vi "filter_logic_chargeupdate.vi"(9 "Filter Specific Constants":T2, 10 "Variables Cluster":T4, 11 "constants cluster":T1={"High Charge Limit"=0, "Low Charge Limit"=0, "Low Velocity Count"=0, "High Velocity Count"=0, "Low Velocity Count"=0, 26666666.59375, "High Mass Limit"=0, "Low Mass Limit"=0}) -> (3 "Output Cluster":T3)   [LabVIEW 2012]
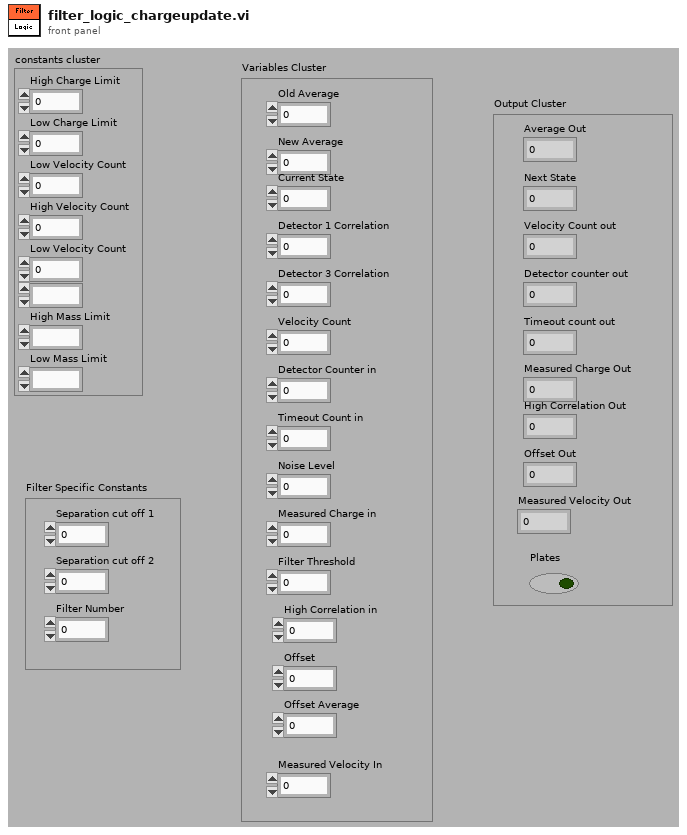
[diagram p1: front panel]
types:
  T1 = cluster{"High Charge Limit":i16, "Low Charge Limit":i16, "Low Velocity Count":i32, "High Velocity Count":i32, "Low Velocity Count":i32, fxp<+,30,25>, "High Mass Limit":i64, "Low Mass Limit":i64}
  T2 = cluster{"Separation cut off 1":i32, "Filter Number":i32, "Separation cut off 2":i32}
  T3 = cluster{"Average Out":i32, "Next State":u8, "Velocity Count out":i32, "Detector counter out":i32, "Timeout count out":u32, "Measured Charge Out":i32, "High Correlation Out":i32, "Plates":bool, "Offset Out":i32, "Measured Velocity Out":i32}
  T4 = cluster{"Old Average":i32, "New Average":i32, "Current State":u8, "Detector 1 Correlation":i32, "Detector 3 Correlation":i32, "Velocity Count":i32, "Detector Counter in":i32, "Timeout Count in":i32, "Noise Level":i32, "Measured Charge in":i32, "Filter Threshold":i32, "High Correlation in":i32, "Offset":i32, "Offset Average":i32, "Measured Velocity In":i32}
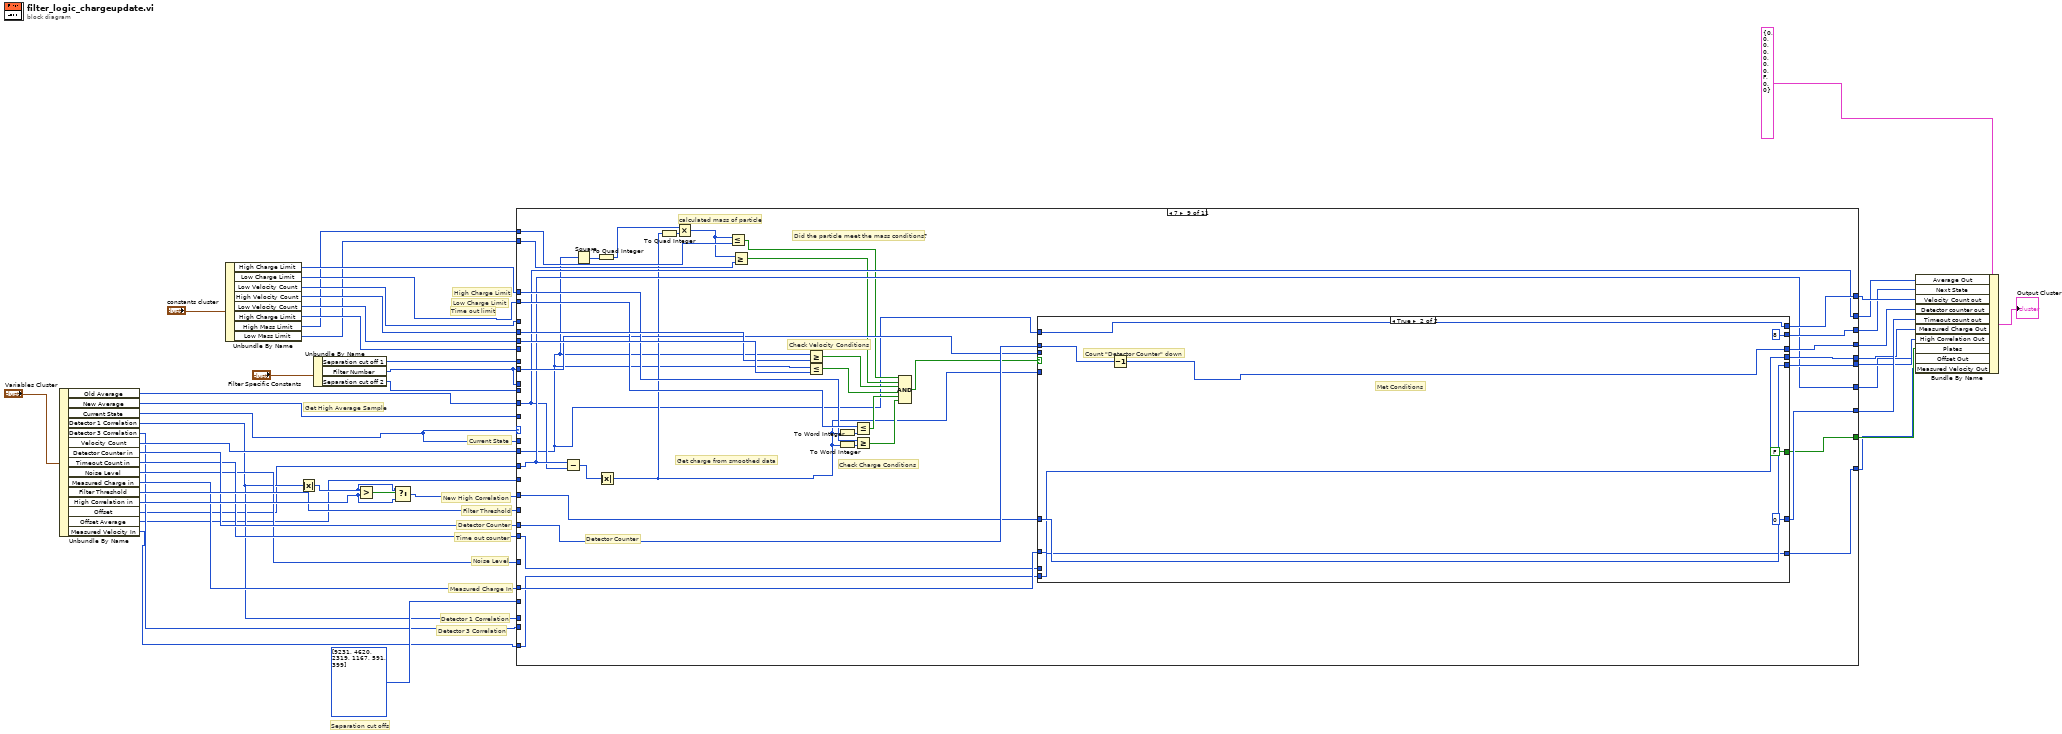
[diagram p0: block diagram]
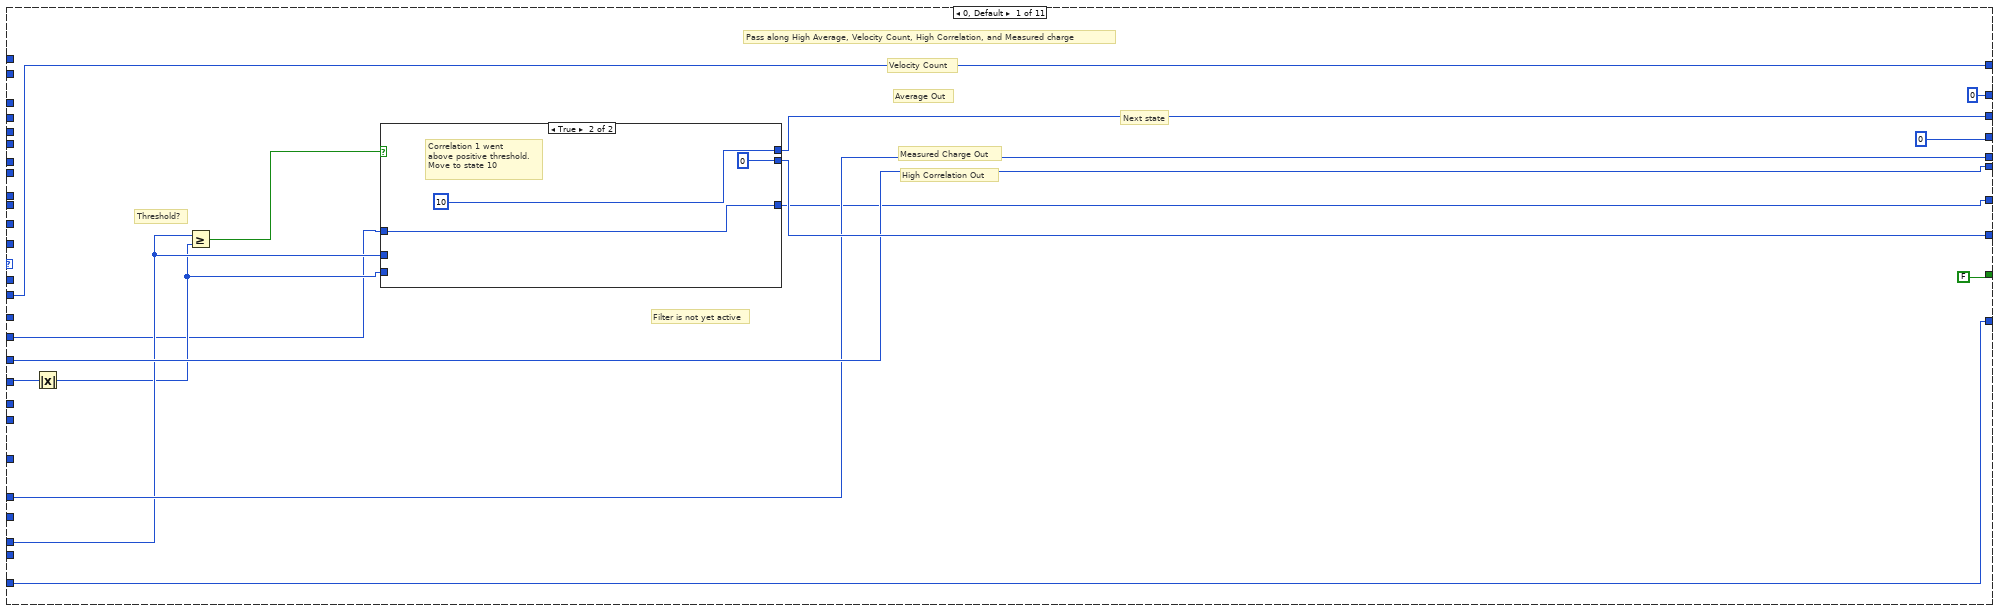
[diagram p2: hidden frame]
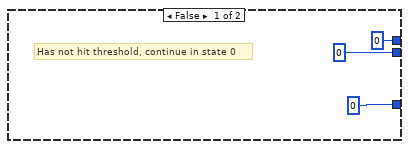
[diagram p3: hidden frame]
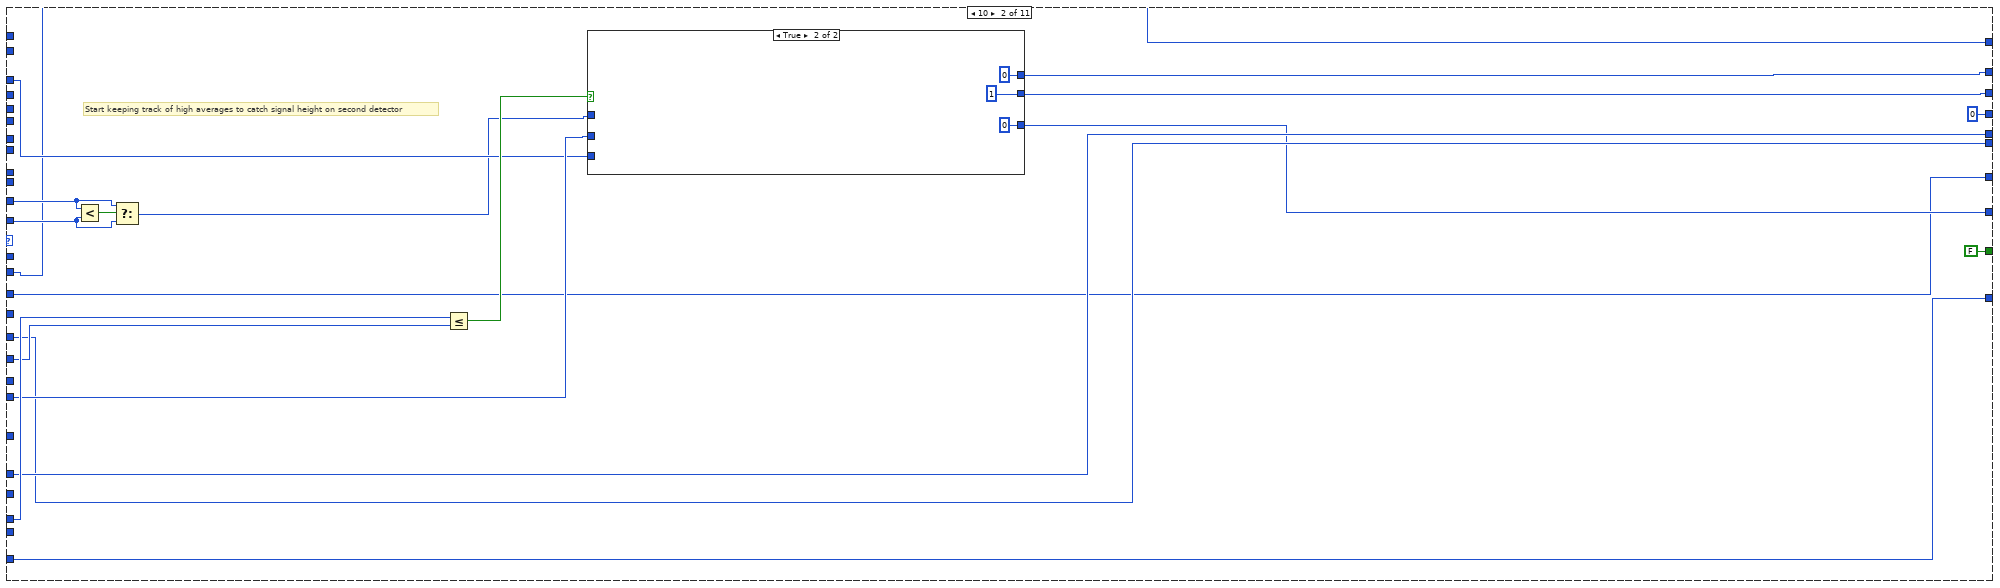
[diagram p4: hidden frame]
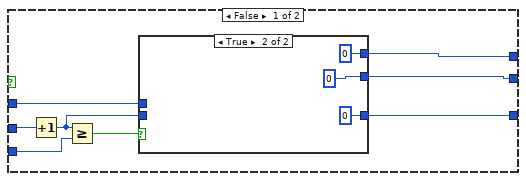
[diagram p5: hidden frame]
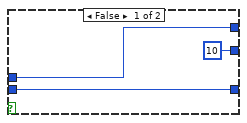
[diagram p6: hidden frame]
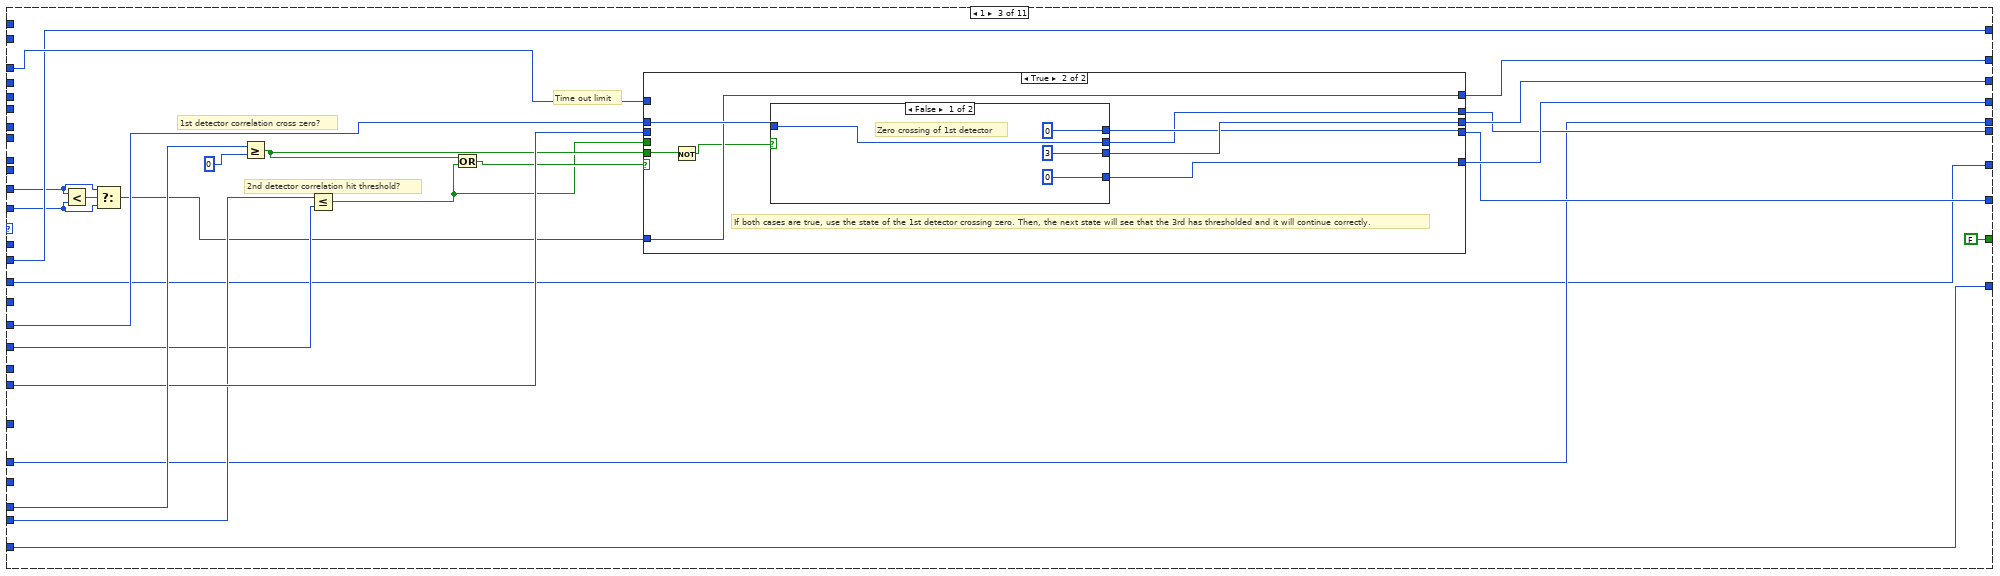
[diagram p7: hidden frame]
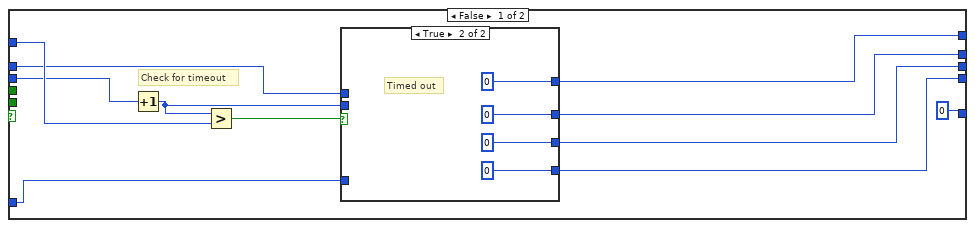
[diagram p8: hidden frame]
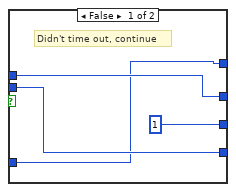
[diagram p9: hidden frame]
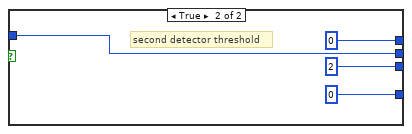
[diagram p10: hidden frame]
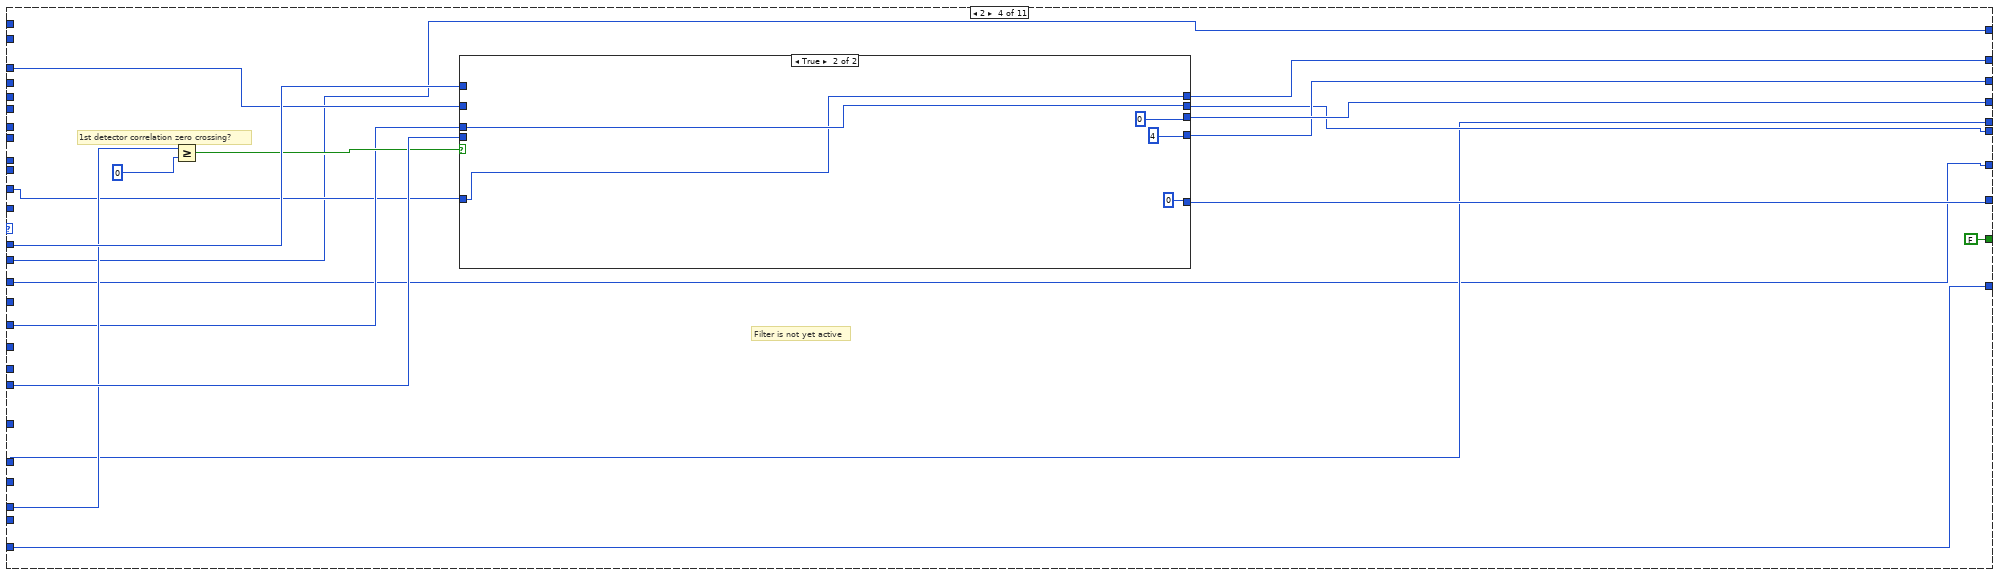
[diagram p11: hidden frame]
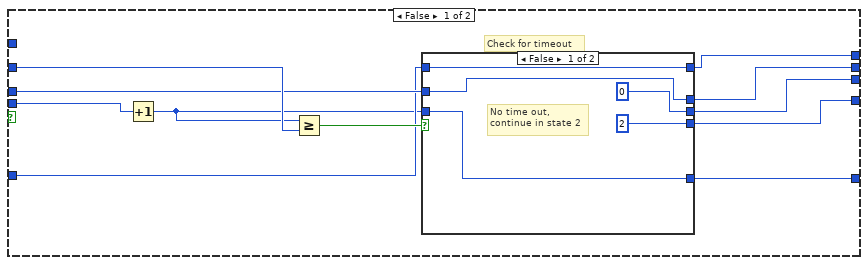
[diagram p12: hidden frame]
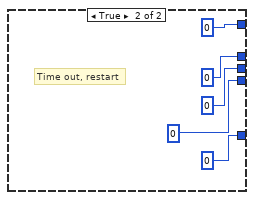
[diagram p13: hidden frame]
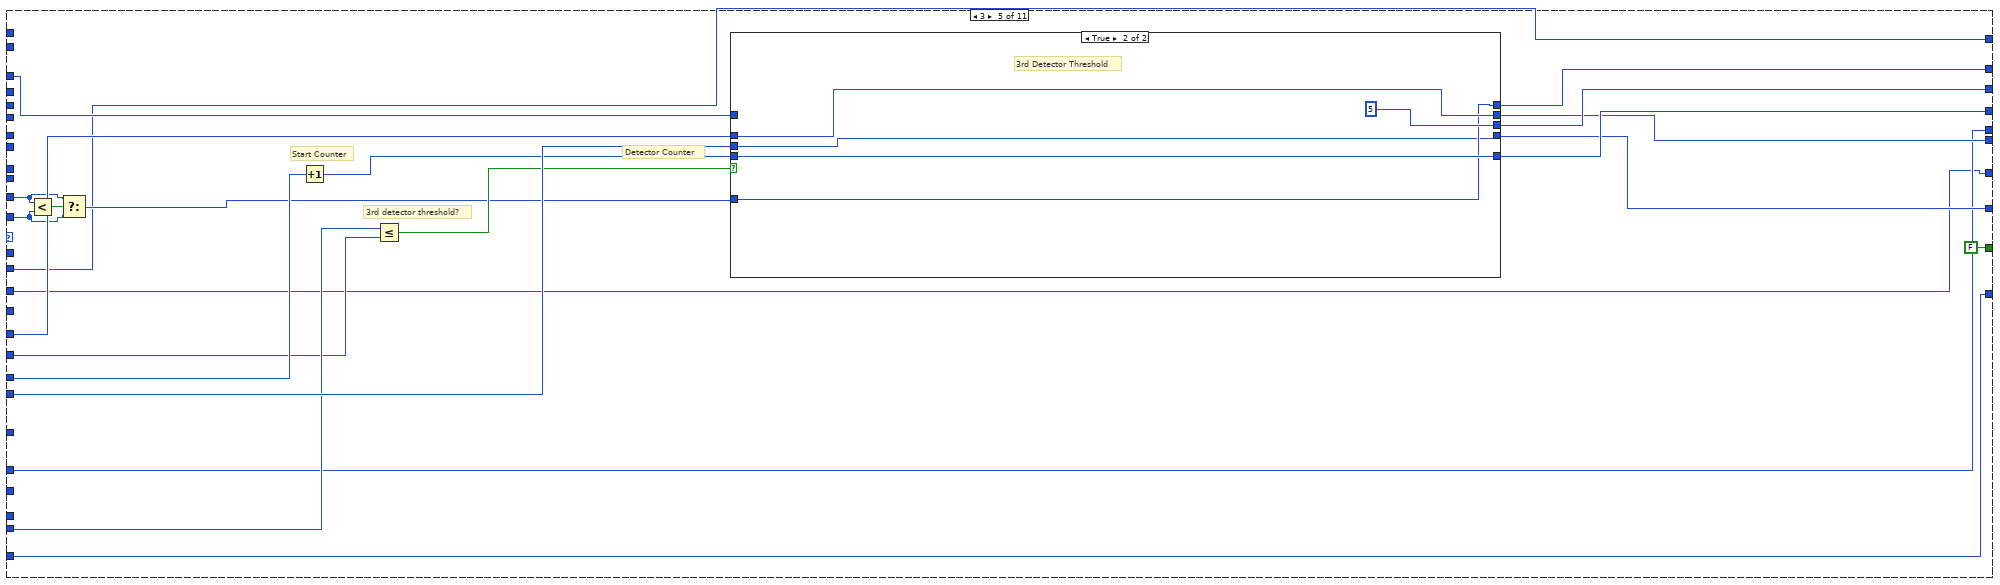
[diagram p14: hidden frame]
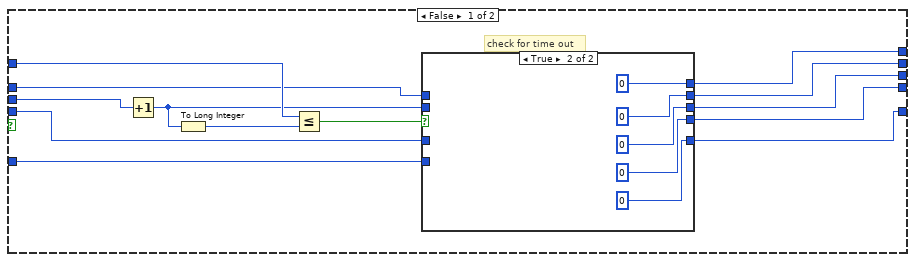
[diagram p15: hidden frame]
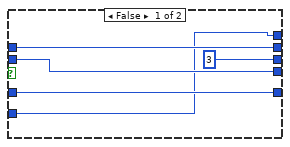
[diagram p16: hidden frame]
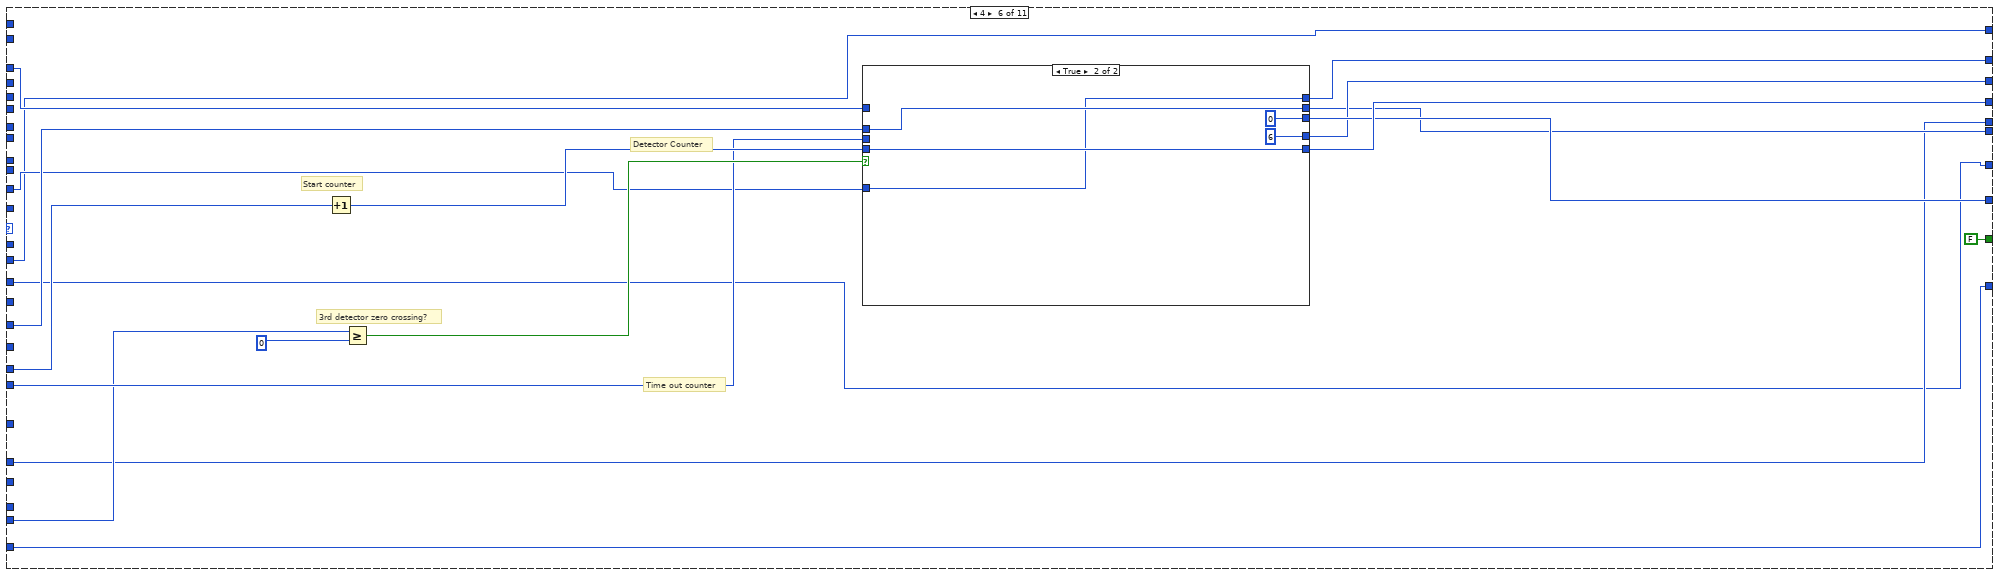
[diagram p17: hidden frame]
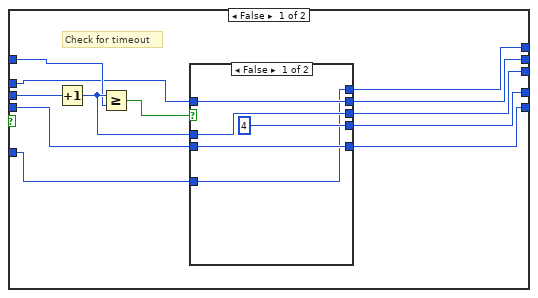
[diagram p18: hidden frame]
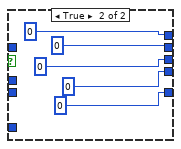
[diagram p19: hidden frame]
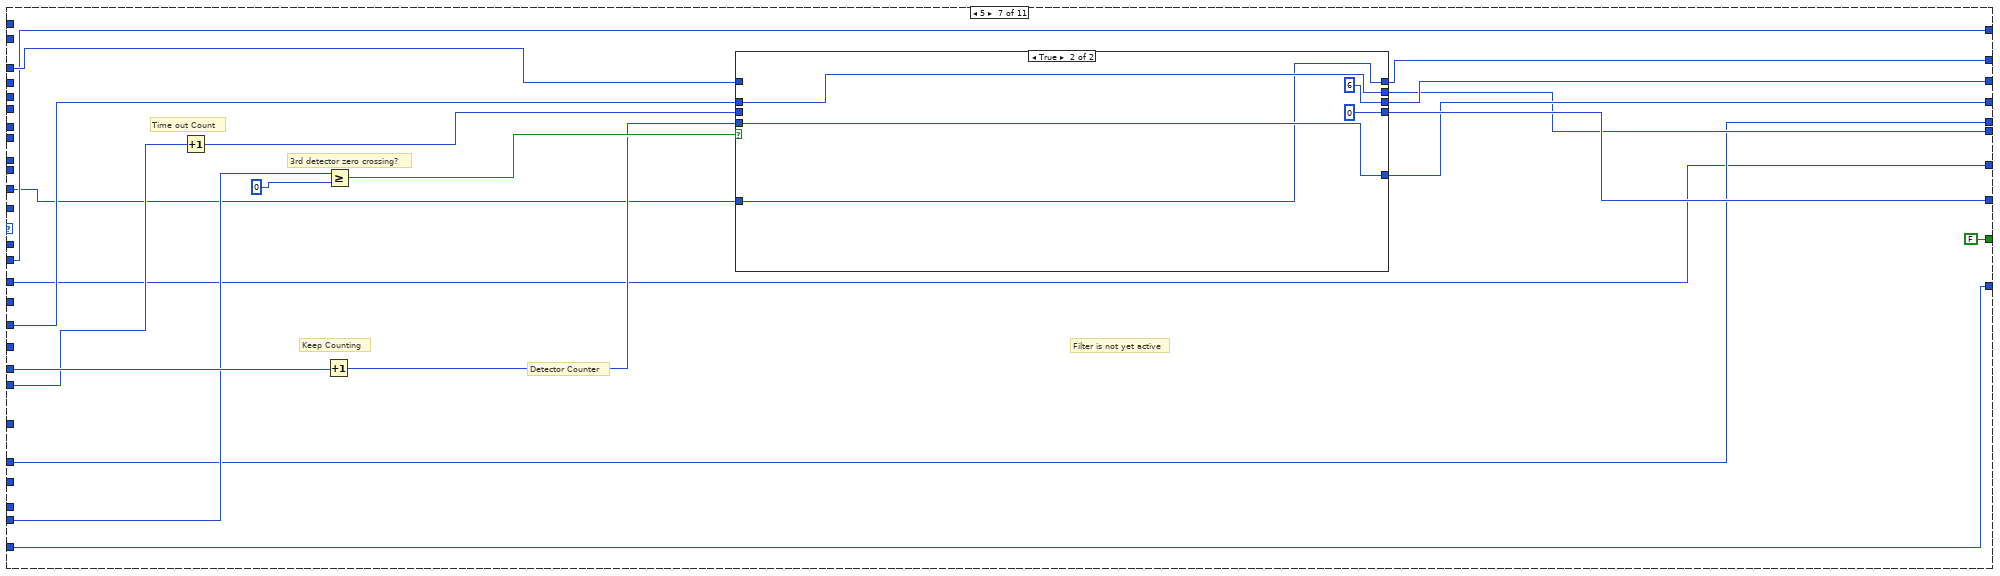
[diagram p20: hidden frame]
diagram:
  # "Detector 3 Correlation"
  # "Detector 1 Correlation"
  # "Separation cut offs"
  # "Measured Charge In"
  # "Noise Level"
  # "Time out counter"
  # "Detector Counter"
  # "Filter Threshold"
  # "New High Correlation"
  # "Current State"
  # "Get High Average Sample"
  # "Time out limit"
  # "Low Charge Limit"
  # "High Charge Limit"
  n1 = Unbundle By Name("Variables Cluster") -> ("Old Average"=w17:i32, "New Average"=w16:i32, "Current State"=w39:u8, "Detector 1 Correlation"=w27:i32, "Detector 3 Correlation"=w26:i32, "Velocity Count"=w38:i32, "Detector Counter in"=w32:i32, "Timeout Count in"=w31:i32, "Noise Level"=w30:i32, "Measured Charge in"=w29:i32, "Filter Threshold"=w33:i32, "High Correlation in"=w34:i32, "Offset"=w15:i32, "Offset Average"=w14:i32, "Measured Velocity In"=w10:i32)
  n2 = Unbundle By Name("constants cluster") -> ("High Charge Limit"=w9:i16, "Low Charge Limit"=w8:i16, "Low Velocity Count"=w7:i32, "High Velocity Count"=w6:i32, "Low Velocity Count"=w5:i32, "High Charge Limit"=w4:i16, "High Mass Limit"=w3:i64, "Low Mass Limit"=w2:i64)
  n3 = Absolute Value(x=w27) -> (abs(x)=w35:i32)
  n4 = Unbundle By Name("Filter Specific Constants") -> ("Separation cut off 1"=w43:i32, "Filter Number"=w42:i32, "Separation cut off 2"=w41:i32)
  n5 = Greater?(x=w35, y=w34) -> (0:w36:bool)
  n6 = Select(t=w35, s=w36, f=w34) -> (s? t:f=w37:i32)
  n7 = case shown="7" w39 {
    tunnel: w27 -> [w52 w82 w126 w173 _ _ _ _ _ _ _]
    tunnel: w26 -> [_ _ w115 _ w219 w266 w311 _ _ _ _]
    tunnel: w33 -> [w50 w81 w114 _ w218 _ _ _ _ _ _]
    tunnel: w32 -> [_ _ _ _ w221 w274 w320 w354 w482 w515 w549]
    tunnel: [0 0 w124 w179 w227 w272 w313 w366 w481 w511 w545] -> w23
    tunnel: [w60 w79 w123 w178 w226 w269 w316 w363 w480 w513 w546] -> w19
    tunnel: w39 -> [_ _ _ w177 _ _ _ _ _ _ _]
    tunnel: w38 -> [w56 w74 w116 w163 w207 w257 w312 w364 w445 w516 w543]
    tunnel: w7 -> [_ w77 w122 w176 w224 w267 w317 _ _ _ _]
    tunnel: w31 -> [_ w78 w121 w175 w225 w268 w319 _ w469 _ _]
    tunnel: [w59 w69 w120 w174 w223 w270 w315 u32 0 w468 u32 0 ("Timeout Count in") u32 0] -> w22
    tunnel: w5 -> [_ _ _ _ _ _ _ _ w479 _ _]
    tunnel: w6 -> [_ _ _ _ _ _ _ _ w478 _ _]
    tunnel: [w56 w74 w116 w163 w207 w257 w312 w365 w477 w512 w543] -> w25
    tunnel: i32[] [9231, 4620, 2319, 1167, 591, 399] -> [_ _ _ _ _ _ _ w357 _ _ _]
    tunnel: w8 -> [_ _ _ _ _ _ _ _ w476 _ _]
    tunnel: w9 -> [_ _ _ _ _ _ _ _ w475 _ _]
    tunnel: w37 -> [w55 w71 w113 w170 w217 w260 w309 w361 w474 w509 w541]
    tunnel: w30 -> [_ _ _ _ _ _ _ _ _ _ _]
    tunnel: [w55 w71 w112 w169 w216 w264 w308 w362 w473 w509 w542] -> w20
    tunnel: w29 -> [w54 w72 w111 w168 w215 w263 w307 w360 w472 w504 w537]
    tunnel: [w54 w72 w111 w168 w215 w263 w307 w360 w471 w505 w537] -> w21
    tunnel: [0 ("Old Average In") w75 w110 w167 w214 w262 w306 w359 w459 w501 0 ("Old Average In")] -> w24
    tunnel: w43 -> [_ _ _ _ _ _ _ w356 _ _ _]
    tunnel: w42 -> [_ _ _ _ _ _ _ w358 _ _ _]
    tunnel: w42 -> [_ _ _ _ _ _ _ w352 w470 w514 w540]
    tunnel: w41 -> [_ _ _ _ _ _ _ w355 _ _ _]
    tunnel: [FALSE FALSE ("Data") FALSE FALSE FALSE FALSE FALSE FALSE w465 w508 w536] -> w18
    tunnel: w17 -> [_ w84 w107 w165 w211 w259 w304 w350 w459 w501 _]
    tunnel: w16 -> [_ w83 w106 _ w210 _ _ _ _ _ _]
    tunnel: w15 -> [_ w68 w104 w164 w208 w258 w303 w349 w460 w500 _]
    tunnel: w14 -> [w47 _ _ _ _ _ _ _ _ _ _]
    tunnel: [w48 w68 w104 w164 w208 w258 w303 w349 w460 w500 0 ("Offset")] -> w13
    tunnel: [w46 w67 w103 w162 w206 w256 w302 w348 w462 w506 w534] -> w11
    tunnel: w10 -> [w46 w67 w103 w162 w206 w256 w302 w348 w461 w507 w534]
    tunnel: w4 -> [_ _ _ _ _ _ _ _ _ _ _]
    tunnel: w3 -> [_ _ _ _ _ _ _ _ w458 _ _]
    tunnel: w2 -> [_ _ _ _ _ _ _ _ w457 _ _]
    frame 0, Default {
      # "Filter is not yet active"
      # "High Correlation Out"
      # "Measured Charge Out"
      # "Next state"
      # "Average Out"
      # "Velocity Count"
      # "Pass along High Average, Velocity Count, High Correlation, and Measured charge"
      # "Threshold?"
      n8 = Absolute Value(x=w50) -> (abs(x)=w49:i32)
      n9 = Greater Or Equal?(x=w52, y=w49) -> (x >= y?=w57:bool)
      n10 = case shown="True" w57 {
        tunnel: [u8 0 u8 10] -> w60
        tunnel: [u32 0 u32 0] -> w59
        tunnel: w52 -> [_ _]
        tunnel: w49 -> [_ _]
        tunnel: [0 w64] -> w48
        tunnel: w47 -> [_ w64]
        frame False {
          # "Has not hit threshold, continue in state 0"
        }
        frame True {
          # "Correlation 1 went\nabove positive threshold.\nMove to state 10"
        }
      }
    }
    frame 10 {
      # "Start keeping track of high averages to catch signal height on second detector"
      n11 = Less?(x=w84, y=w83) -> (x < y?=w85:bool)
      n12 = Select(t=w84, s=w85, f=w83) -> (s? t:f=w76:i32)
      n13 = Less Or Equal?(x=w82, y=w81) -> (x <= y?=w80:bool)
      n14 = case shown="True" w80 {
        tunnel: [w91 u8 1] -> w79
        tunnel: w78 -> [w88 _]
        tunnel: w77 -> [w93 _]
        tunnel: w76 -> [w90 _]
        tunnel: [w89 0 ("New Average")] -> w75
        tunnel: [w86 0] -> w69
        frame False {
          n15 = Increment(x=w88) -> (x+1=w87:i32)
          n16 = Greater Or Equal?(x=w87, y=w93) -> (x >= y?=w92:bool)
          n17 = case shown="True" w92 {
            tunnel: [u8 10 u8 0] -> w91
            tunnel: w90 -> [w96 _]
            tunnel: [w96 0 ("New Average")] -> w89
            tunnel: w87 -> [w94 _]
            tunnel: [w94 0] -> w86
            frame False {
            }
            frame True {
            }
          }
        }
        frame True {
        }
      }
    }
    frame 1 {
      # "Time out limit"
      # "2nd detector correlation hit threshold?"
      # "1st detector correlation cross zero?"
      n18 = Less?(x=w107, y=w106) -> (x < y?=w108:bool)
      n19 = Select(t=w107, s=w108, f=w106) -> (s? t:f=w105:i32)
      n20 = Greater Or Equal?(x=w126, y=0) -> (x >= y?=w118:bool)
      n21 = Less Or Equal?(x=w115, y=w114) -> (x <= y?=w117:bool)
      n22 = Or(x=w118, y=w117) -> (x .or. y?=w119:bool)
      n23 = case shown="True" w119 {
        tunnel: [0 w152] -> w124
        tunnel: [w135 w153] -> w123
        tunnel: w122 -> [w137 _]
        tunnel: w121 -> [w134 _]
        tunnel: [w133 w151] -> w120
        tunnel: w118 -> [_ w147]
        tunnel: w117 -> [_ _]
        tunnel: w113 -> [w131 w150]
        tunnel: [w130 w149] -> w112
        tunnel: [w129 w148] -> w110
        tunnel: w105 -> [w127 w148]
        frame False {
          # "Check for timeout"
          n24 = Increment(x=w134) -> (x+1=w128:i32)
          n25 = Greater?(x=w128, y=w137) -> (0:w136:bool)
          n26 = case shown="True" w136 {
            tunnel: [u8 1 u8 0] -> w135
            tunnel: w128 -> [w140 _]
            tunnel: [w140 u32 0] -> w133
            tunnel: w131 -> [w139 _]
            tunnel: [w139 0 ("High Correlation In")] -> w130
            tunnel: [w138 0 ("Old Average In")] -> w129
            tunnel: w127 -> [w138 _]
            frame False {
              # "Didn't time out, continue"
            }
            frame True {
              # "Timed out"
            }
          }
        }
        frame True {
          # "If both cases are true, use the state of the 1st detector crossing zero. Then, the next state will see that the 3rd has thresholded and it will continue correctly."
          n27 = Not(x=w147) -> (.not. x?=w146:bool)
          n28 = case shown="False" w146 {
            tunnel: [u8 3 u8 2] -> w153
            tunnel: [0 0] -> w152
            tunnel: [u32 0 u32 0] -> w151
            tunnel: w150 -> [w154 w158]
            tunnel: [w154 w158] -> w149
            frame False {
              # "Zero crossing of 1st detector"
            }
            frame True {
              # "second detector threshold"
            }
          }
        }
      }
    }
    frame 2 {
      # "Filter is not yet active"
      # "1st detector correlation zero crossing?"
      n29 = Greater Or Equal?(x=w173, y=0) -> (x >= y?=w171:bool)
      n30 = case shown="True" w171 {
        tunnel: [w185 0] -> w179
        tunnel: [w189 u8 4] -> w178
        tunnel: w177 -> [_ _]
        tunnel: w176 -> [w188 _]
        tunnel: w175 -> [w186 _]
        tunnel: [w187 u32 0] -> w174
        tunnel: w170 -> [w184 w202]
        tunnel: [w183 w202] -> w169
        tunnel: [w182 w201] -> w167
        tunnel: w165 -> [w181 w201]
        frame False {
          # "Check for timeout"
          n31 = Increment(x=w186) -> (x+1=w180:i32)
          n32 = Greater Or Equal?(x=w180, y=w188) -> (x >= y?=w190:bool)
          n33 = case shown="False" w190 {
            tunnel: [u8 2 u8 0] -> w189
            tunnel: w180 -> [w195 _]
            tunnel: [w195 u32 0] -> w187
            tunnel: [0 0] -> w185
            tunnel: w184 -> [w192 _]
            tunnel: [w192 0 ("High Correlation In")] -> w183
            tunnel: [w191 0 ("Old Average In")] -> w182
            tunnel: w181 -> [w191 _]
            frame False {
              # "No time out, \ncontinue in state 2"
            }
            frame True {
              # "Time out, restart"
            }
          }
        }
        frame True {
        }
      }
    }
    frame 3 {
      # "3rd detector threshold?"
      # "Start Counter"
      # "Detector Counter"
      n34 = Less?(x=w211, y=w210) -> (x < y?=w212:bool)
      n35 = Select(t=w211, s=w212, f=w210) -> (s? t:f=w209:i32)
      n36 = Increment(x=w221) -> (x+1=w220:i32)
      n37 = Less Or Equal?(x=w219, y=w218) -> (x <= y?=w222:bool)
      n38 = case shown="True" w222 {
        tunnel: w220 -> [w235 w255]
        tunnel: [w234 w255] -> w227
        tunnel: [w237 u8 5] -> w226
        tunnel: w225 -> [w233 w251]
        tunnel: w224 -> [w240 _]
        tunnel: [w236 w251] -> w223
        tunnel: w217 -> [w231 w253]
        tunnel: [w230 w253] -> w216
        tunnel: [w229 w252] -> w214
        tunnel: w209 -> [w228 w252]
        frame False {
          # "check for time out"
          n39 = Increment(x=w233) -> (x+1=w232:i32)
          n40 = To Long Integer(number=w232) -> (32bit integer=w239:i32)
          n41 = Less Or Equal?(x=w240, y=w239) -> (x <= y?=w238:bool)
          n42 = case shown="True" w238 {
            tunnel: [u8 3 u8 0] -> w237
            tunnel: w232 -> [w244 _]
            tunnel: [w244 u32 0] -> w236
            tunnel: w235 -> [w243 _]
            tunnel: [w243 0] -> w234
            tunnel: w231 -> [w242 _]
            tunnel: [w242 0 ("High Correlation In")] -> w230
            tunnel: [w241 0 ("Old Average In")] -> w229
            tunnel: w228 -> [w241 _]
            frame False {
            }
            frame True {
            }
          }
        }
        frame True {
          # "3rd Detector Threshold"
        }
      }
    }
    frame 4 {
      # "Time out counter"
      # "3rd detector zero crossing?"
      # "Start counter"
      # "Detector Counter"
      n43 = Increment(x=w274) -> (x+1=w271:i32)
      n44 = Greater Or Equal?(x=w266, y=0) -> (x >= y?=w273:bool)
      n45 = case shown="True" w273 {
        tunnel: [w279 w301] -> w272
        tunnel: w271 -> [w280 w301]
        tunnel: [w282 u32 0] -> w270
        tunnel: [w284 u8 6] -> w269
        tunnel: w268 -> [w286 _]
        tunnel: w267 -> [w281 _]
        tunnel: w260 -> [w278 w298]
        tunnel: [w277 w298] -> w264
        tunnel: [w276 w297] -> w262
        tunnel: w259 -> [w275 w297]
        frame False {
          # "Check for timeout"
          n46 = Increment(x=w286) -> (x+1=w283:i32)
          n47 = Greater Or Equal?(x=w283, y=w281) -> (x >= y?=w285:bool)
          n48 = case shown="False" w285 {
            tunnel: [u8 4 u8 0] -> w284
            tunnel: w283 -> [w290 _]
            tunnel: [w290 u32 0] -> w282
            tunnel: w280 -> [w289 _]
            tunnel: [w289 0] -> w279
            tunnel: w278 -> [w288 _]
            tunnel: [w288 0 ("High Correlation In")] -> w277
            tunnel: [w287 0 ("Old Average In")] -> w276
            tunnel: w275 -> [w287 _]
            frame False {
            }
            frame True {
            }
          }
        }
        frame True {
        }
      }
    }
    frame 5 {
      # "Filter is not yet active"
      # "Time out Count"
      # "3rd detector zero crossing?"
      # "Keep Counting"
      # "Detector Counter"
      n49 = Increment(x=w319) -> (x+1=w318:i32)
      n50 = Increment(x=w320) -> (x+1=w314:i32)
      n51 = Greater Or Equal?(x=w311, y=0) -> (x >= y?=w321:bool)
      n52 = case shown="True" w321 {
        tunnel: w318 -> [w328 _]
        tunnel: w317 -> [w332 _]
        tunnel: [w330 u8 6] -> w316
        tunnel: [w329 u32 0] -> w315
        tunnel: w314 -> [w327 w345]
        tunnel: [w326 w345] -> w313
        tunnel: w309 -> [w324 w344]
        tunnel: [w325 w344] -> w308
        tunnel: [w323 w343] -> w306
        tunnel: w304 -> [w322 w343]
        frame False {
          # "Check for timeout"
          n53 = Greater Or Equal?(x=w328, y=w332) -> (x >= y?=w331:bool)
          n54 = case shown="False" w331 {
            tunnel: [u8 5 u8 0] -> w330
            tunnel: [w336 u32 0] -> w329
            tunnel: w328 -> [w336 _]
            tunnel: w327 -> [w335 _]
            tunnel: [w335 0] -> w326
            tunnel: [w334 0 ("High Correlation In")] -> w325
            tunnel: w324 -> [w334 _]
            tunnel: [w333 0 ("Old Average In")] -> w323
            tunnel: w322 -> [w333 _]
            frame False {
            }
            frame True {
            }
          }
        }
        frame True {
        }
      }
    }
    frame 6 {
      # "Does the velocity of this particle most closely match this filter?"
      # "Detector Counter"
      n55 = case shown="4" w352 {
        tunnel: w357 -> [w375 w381 w385 w394 w404 w412 w421 w431]
        tunnel: w356 -> [w374 w380 w384 w393 w402 w411 w420 w430]
        tunnel: w355 -> [w373 _ w386 w395 w403 w413 w422 _]
        tunnel: w354 -> [w371 w379 w383 w392 w401 w410 w419 w428]
        tunnel: [w370 w377 w382 w391 w400 w409 w418 w427] -> w353
        frame 0, Default {
          n56 = Index Array(array=w375, index=w374) -> (element=w372:i32)
          n57 = Index Array(array=w375, index=w373) -> (element=w376:i32)
          n58 = Greater Or Equal?(x=w371, y=w376) -> (x >= y?=w369:bool)
          n59 = Less?(x=w371, y=w372) -> (x < y?=w368:bool)
          n60 = And(x=w369, y=w368) -> (x .and. y?=w370:bool)
        }
        frame 1 {
          n61 = Index Array(array=w381, index=w380) -> (element=w378:i32)
          n62 = Greater Or Equal?(x=w379, y=w378) -> (x >= y?=w377:bool)
        }
        frame 2 {
          n63 = Index Array(array=w385, index=w384) -> (element=w388:i32)
          n64 = Index Array(array=w385, index=w386) -> (element=w387:i32)
          n65 = Greater Or Equal?(x=w383, y=w387) -> (x >= y?=w389:bool)
          n66 = Less?(x=w383, y=w388) -> (x < y?=w390:bool)
          n67 = And(x=w389, y=w390) -> (x .and. y?=w382:bool)
        }
        frame 3 {
          n68 = Index Array(array=w394, index=w393) -> (element=w397:i32)
          n69 = Index Array(array=w394, index=w395) -> (element=w396:i32)
          n70 = Greater Or Equal?(x=w392, y=w396) -> (x >= y?=w398:bool)
          n71 = Less?(x=w392, y=w397) -> (x < y?=w399:bool)
          n72 = And(x=w398, y=w399) -> (x .and. y?=w391:bool)
        }
        frame 4 {
          # "3"
          # "2"
          n73 = Index Array(array=w404, index=w402) -> (element=w406:i32)
          n74 = Index Array(array=w404, index=w403) -> (element=w405:i32)
          n75 = Greater Or Equal?(x=w401, y=w405) -> (x >= y?=w407:bool)
          n76 = Less?(x=w401, y=w406) -> (x < y?=w408:bool)
          n77 = And(x=w407, y=w408) -> (x .and. y?=w400:bool)
        }
        frame 5 {
          n78 = Index Array(array=w412, index=w411) -> (element=w415:i32)
          n79 = Index Array(array=w412, index=w413) -> (element=w414:i32)
          n80 = Greater Or Equal?(x=w410, y=w414) -> (x >= y?=w416:bool)
          n81 = Less?(x=w410, y=w415) -> (x < y?=w417:bool)
          n82 = And(x=w416, y=w417) -> (x .and. y?=w409:bool)
        }
        frame 6 {
          n83 = Index Array(array=w421, index=w420) -> (element=w425:i32)
          n84 = Index Array(array=w421, index=w422) -> (element=w426:i32)
          n85 = Greater Or Equal?(x=w419, y=w426) -> (x >= y?=w424:bool)
          n86 = Less?(x=w419, y=w425) -> (x < y?=w423:bool)
          n87 = And(x=w424, y=w423) -> (x .and. y?=w418:bool)
        }
        frame 7 {
          n88 = Index Array(array=w431, index=w430) -> (element=w429:i32)
          n89 = Less?(x=w428, y=w429) -> (x < y?=w427:bool)
        }
      }
      n90 = case shown="True" w353 {
        tunnel: [0 w442] -> w366
        tunnel: w354 -> [_ w441]
        tunnel: [w436 w441] -> w365
        tunnel: w364 -> [w436 _]
        tunnel: [u8 0 u8 7] -> w363
        tunnel: [0 ("High Correlation In") w439] -> w362
        tunnel: w361 -> [_ w439]
        tunnel: [0 ("Old Average In") w438] -> w359
        tunnel: w358 -> [_ _]
        tunnel: w350 -> [_ w438]
        frame False {
          # "Incorrect filter, restart"
        }
        frame True {
          (unwired) fxp<+,31,3> 7.340293329209089
          # "Use this number for 3rd detector"
          # "Filter is now active"
          # "Number of cycles to wait until\nopening the plates"
          # "This is applying a multiplier, which is derived from the ratio of lengths of\ndet3 to deflection plates vs. det1 to det3. It includes 15 cm\nof slop, as well as -1.666 detector length, since a signal that is perfectly\nmatched to a filter will have its second zero crossing 1 and 2/3 detector \nlength away from the edge of the 3rd detector"
          # "Correct filter\nCalculate \"wait\" number of cycles"
          n91 = To Fixed-Point(number=w441) -> (fixed-point=w444:fxp<+/-,32,32>)  [unwired: 1 in]
          n92 = Multiply(x=w444, y=fxp<+,22,1> 1.636110782623291) -> (x*y=w443:fxp<+/-,54,33>)
          n93 = To Long Integer(number=w443) -> (32bit integer=w442:i32)
        }
      }
    }
    frame 7 {
      # "Did the particle meet the mass conditions?"
      # "calculated mass of particle"
      # "Get charge from smoothed data"
      # "Check Velocity Conditions"
      # "Check Charge Conditions"
      # "Detector Counter"
      n94 = Subtract(x=w460, y=w459) -> (x-y=w464:i32)
      n95 = Square(x=w445) -> (x^2=w449:i32)
      n96 = To Quad Integer(1:w449) -> (0:w448:i64)
      n97 = Absolute Value(x=w464) -> (abs(x)=w446:i32)
      n98 = To Quad Integer(1:w446) -> (0:w447:i64)
      n99 = Multiply(x=w448, y=w447) -> (x*y=w450:i64)
      n100 = Less Or Equal?(x=w450, y=w458) -> (x <= y?=w451:bool)
      n101 = Greater Or Equal?(x=w450, y=w457) -> (x >= y?=w452:bool)
      n102 = Greater Or Equal?(x=w445, y=w478) -> (x >= y?=w453:bool)
      n103 = Less Or Equal?(x=w445, y=w479) -> (x <= y?=w454:bool)
      n104 = To Word Integer(number=w446) -> (16bit integer=w467:i16)
      n105 = To Word Integer(number=w446) -> (16bit integer=w466:i16)
      n106 = Less Or Equal?(x=w476, y=w467) -> (x <= y?=w455:bool)
      n107 = Greater Or Equal?(x=w475, y=w466) -> (x >= y?=w456:bool)
      n108 = Compound Arithmetic op=AND(w451, w452, w453, w454, w455, w456) -> (w463:bool)
      n109 = case shown="True" w463 {
        tunnel: w482 -> [_ w499]
        tunnel: w445 -> [w489 w493]
        tunnel: [0 w497] -> w481
        tunnel: [u8 0 u8 8] -> w480
        tunnel: [w489 w493] -> w477
        tunnel: w474 -> [_ w498]
        tunnel: [0 ("High Correlation In") w498] -> w473
        tunnel: w472 -> [w486 w491]
        tunnel: w446 -> [_ _]
        tunnel: [w486 w491] -> w471
        tunnel: w470 -> [_ _]
        tunnel: w469 -> [_ _]
        tunnel: [u32 0 ("Timeout Count in") 0 ("Timeout Count in")] -> w468
        tunnel: [FALSE ("Data") FALSE ("Data")] -> w465
        tunnel: [w483 w492] -> w462
        tunnel: w461 -> [w483 w492]
        frame False {
          # "Correct filter, but wrong velocity and/or charge."
          # "Did not meet conditions, restart"
        }
        frame True {
          # "Met Conditions"
          # "Count \"Detector Counter\" down"
          n110 = Decrement(x=w499) -> (x-1=w497:i32)
        }
      }
    }
    frame 8 {
      # "Met Conditions, declare that this filter is active and count down until opening the plates"
      # "Count \"Detector Counter\" down"
      # "velocity count"
      n111 = Subtract(x=w500, y=w501) -> (x-y=w503:i32)
      n112 = Absolute Value(x=w503) -> (abs(x)=w502:i32)
      n113 = Decrement(x=w515) -> (x-1=w517:i32)
      n114 = Less Or Equal?(x=w517, y=0) -> (x <= y?=w518:bool)
      n115 = case shown="True" w518 {
        tunnel: [u8 8 u8 9] -> w513
        tunnel: [w525 w532] -> w511
        tunnel: w516 -> [w523 w527]
        tunnel: w517 -> [w525 _]
        tunnel: [w523 w527] -> w512
        tunnel: w514 -> [_ _]
        tunnel: [FALSE ("Data") TRUE ("Data")] -> w508
        tunnel: w507 -> [w521 _]
        tunnel: [w521 w527] -> w506
        tunnel: [w520 w526] -> w505
        tunnel: w504 -> [w520 _]
        tunnel: w502 -> [_ w526]
        frame False {
          # "Counting down to wait to open the plates"
        }
        frame True {
          # "Plates are available so\nallow access to plates"
          # "velocity count"
          # "Number derived from ratio of lengths of plates (w/ 25cm of slop)\n vs. det1 to det3"
          # "clock counts to wait \nuntil close."
          # "Need to open the plates\nhere. Check availablility of plates, and if available, set memory to true to open them"
          n116 = To Fixed-Point(number=w527) -> (fixed-point=w529:fxp<+/-,32,32>)  [unwired: 1 in]
          n117 = Multiply(x=w529, y=fxp<+,18,0> 0.7666587829589844 ("x")) -> (x*y=w533:fxp<+/-,50,32>)
          n118 = To Long Integer(number=w533) -> (32bit integer=w532:i32)
        }
      }
    }
    frame 9 {
      # "Count down and then close plates"
      # "Detector Counter"
      n119 = Decrement(x=w549) -> (x-1=w544:i32)
      n120 = Less Or Equal?(x=w544, y=0) -> (x <= y?=w547:bool)
      n121 = case shown="True" w547 {
        tunnel: [w552 0] -> w545
        tunnel: [u8 9 u8 0] -> w546
        tunnel: w544 -> [w552 _]
        tunnel: w541 -> [w551 _]
        tunnel: [w551 0 ("Noise Level")] -> w542
        tunnel: w540 -> [_ _]
        tunnel: [TRUE ("Data") FALSE ("Data")] -> w536
        frame False {
          # "Count down to wait to close the plates"
        }
        frame True {
          # "Restart"
          # "Close plates here"
        }
      }
    }
  }
  n122 = Bundle By Name(cluster=T3 {"Average Out"=0, "Next State"=0, "Velocity Count out"=0, "Detector counter out"=0, "Timeout count out"=0, "Measured Charge Out"=0, "High Correlation Out"=0, "Plates"=FALSE, "Offset Out"=0, "Measured Velocity Out"=0} ("Output Cluster"), "Average Out"=w24, "Next State"=w19, "Velocity Count out"=w25, "Detector counter out"=w23, "Timeout count out"=w22, "Measured Charge Out"=w21, "High Correlation Out"=w20, "Plates"=w18, "Offset Out"=w13, "Measured Velocity Out"=w11) -> (→"Output Cluster":T3)
